vi "Get Force.vi"(8 "error in (no error)":errorcluster, 11 "Force Sensor in":refnum<class "Force Sensor.lvclass">) -> (0 "error out":errorcluster, 2 "force (V)":dbl, 3 "Force Sensor out":refnum<class "Force Sensor.lvclass">)   [LabVIEW 2020, in "Force Sensor.lvclass"]
uses:
  Force Sensor.lvclass
  Force Sensor.lvclass/Force Sensor.ctl
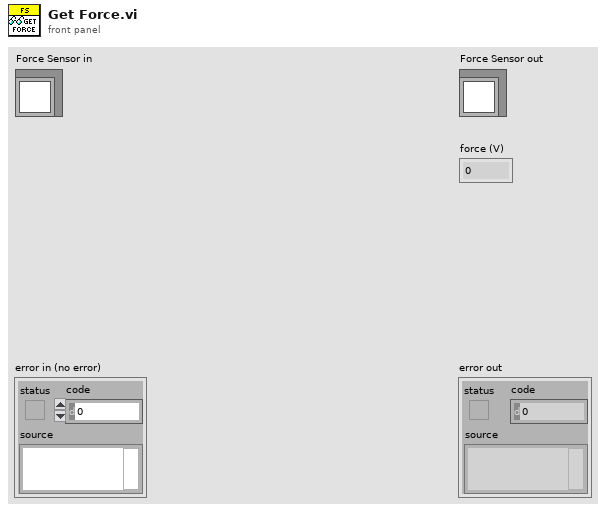
[diagram p1: front panel]
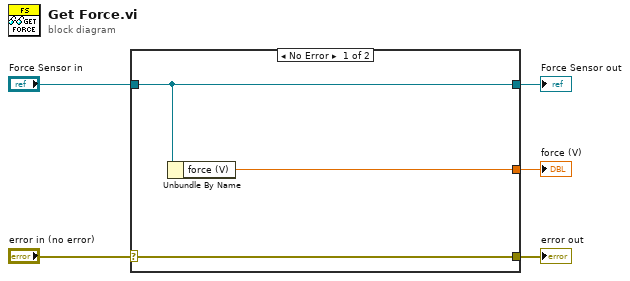
[diagram p0: block diagram]
diagram:
  n1 = case shown="No Error" "error in (no error)" {
    selector: "error in (no error)" -> [w8 w9]
    tunnel: [w8 w9] -> w4
    tunnel: [w7 w10] -> w2
    tunnel: "Force Sensor in" -> [w7 w10]
    tunnel: [w6 _] -> w1
    frame No Error {
      n2 = Unbundle By Name(w7) -> ("force (V)"=w6:dbl)
    }
    frame Error {
    }
  }
  "error out" <- w4
  "Force Sensor out" <- w2
  "force (V)" <- w1
